vi "Relay Control.vi"(8 "error in (no error)":errorcluster, 9 "relay action (Close Relay)":T1=21 items=["Open Relay"=20, "Close Relay"=21], 10 "relay names":string, 11 "instrument handle":refnum<k15>) -> (0 "error out":errorcluster, 3 "instrument handle out":refnum<k15>)   [LabVIEW 2015]
uses:
  <instrlib>/niSwitch/niSwitch.llb/niSwitch Relay Action.ctl
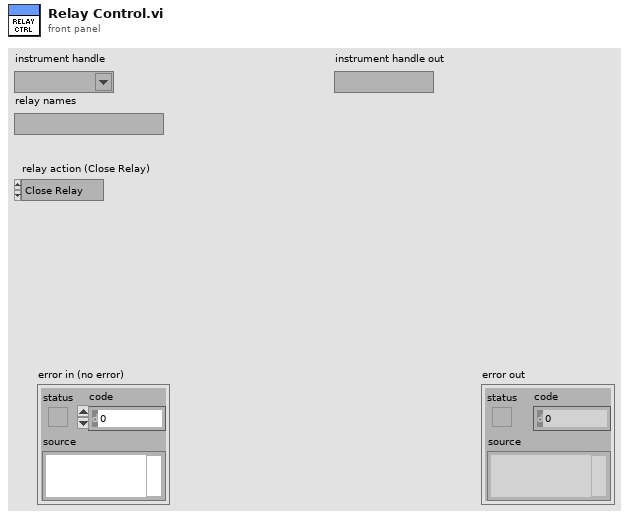
[diagram p1: front panel]
types:
  T1 = typedef "niSwitch Relay Action.ctl" = i32
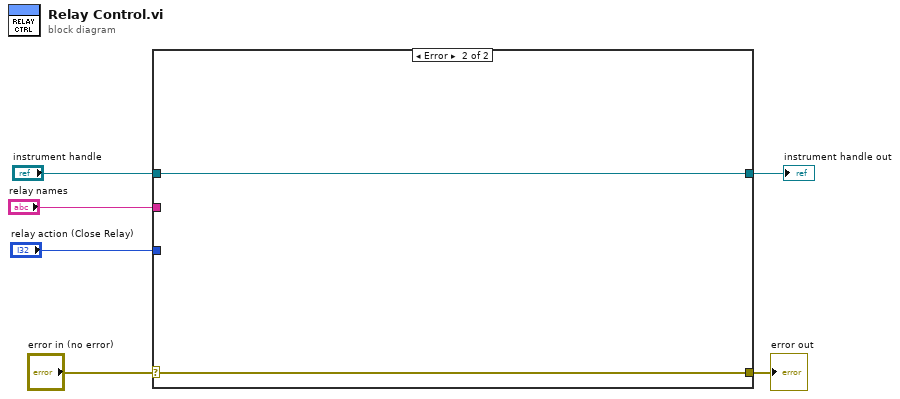
[diagram p0: block diagram]
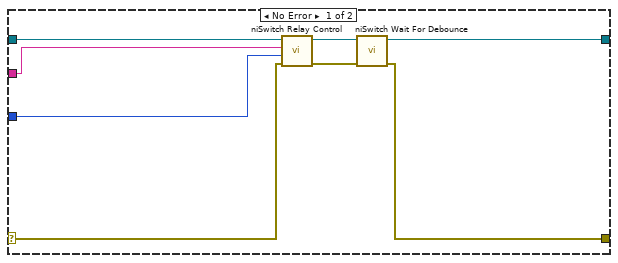
[diagram p2: hidden frame]
diagram:
  n1 = case shown="Error" "error in (no error)" {
    selector: "error in (no error)" -> [w13 w16]
    tunnel: [w10 w16] -> w5
    tunnel: "relay action (Close Relay)" -> [w14 _]
    tunnel: "instrument handle" -> [w9 w15]
    tunnel: [w8 w15] -> w2
    tunnel: "relay names" -> [w7 _]
    frame No Error {
      n2 = call <instrlib>:"niSwitch Relay Control.vi"("error in (no error)"=w13, "relay action (Close Relay)"=w14, "relay names"=w7, "instrument handle"=w9) -> ("error out"=w11:errorcluster, "instrument handle out"=w12:refnum<k15>)  [unwired: 6 in]
      n3 = call <instrlib>:"niSwitch Wait For Debounce.vi"("error in (no error)"=w11, "instrument handle"=w12) -> ("error out"=w10:errorcluster, "instrument handle out"=w8:refnum<k15>)  [unwired: 8 in]
    }
    frame Error {
    }
  }
  "error out" <- w5
  "instrument handle out" <- w2
